vi "WriteComplexeArrayToText.vi"() -> ()   [LabVIEW 2018, in "RW_Protocols.lvlib"]
uses:
  RW_Protocols.lvlib
panel:
  in  "Array":dbl[][](array[numeric])=[[0.0, 0.0, 0.0, 0.0, 0.0, 0.0, 0.0], [0.0, 0.0, 0.0, 0.0, 0.0, 0.0, 0.0], [0.0, 0.0, 0.0, 0.0, 0.0, 0.0, 0.0], [0.0, 0.0, 0.0, 0.0, 0.0, 0.0, 0.0]]
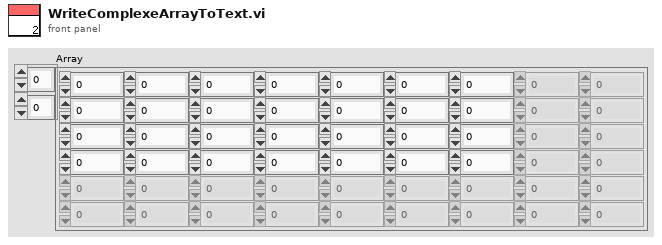
[diagram p1: front panel]
types:
  T1 = enum16{"open", "replace", "create", "open or create", "replace or create", "replace or create with confirmation"}
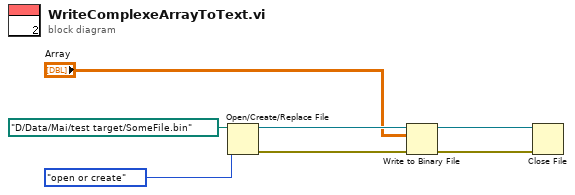
[diagram p0: block diagram]
diagram:
  n1 = Open/Create/Replace File(file path (use dialog)=path "D:/Data/Mai/test target/SomeFile.bin", operation (0:open)=T1."open or create") -> (refnum out=w7:refnum<file>, error out=w5:errorcluster)  [unwired: 4 in, 1 out]
  n2 = Write to Binary File(file (use dialog)=w7, data="Array", error in=w5) -> (refnum out=w6:refnum<file>, error out=w4:errorcluster)  [unwired: 3 in, 1 out]
  n3 = Close File(refnum=w6, error in=w4) -> ()  [unwired: 2 out]
